vi "Average Cycle Bandwidth.vi"(10 "Decimation":u64=1, 11 "Buffer":refnum<class "Buffer.lvclass">) -> (3 "avergage cycle bandwidth":dbl format="%.0g bytes")   [LabVIEW 2017, in "DSF Core.lvlib"]
uses:
  DSF Core.lvlib
  Classes/Buffer/Buffer.lvclass
  C:/Program Files (x86)/National Instruments/LabVIEW 2017/vi.lib/NI/Memory Manager/Classes/Pointer/Pointer.lvclass
  <vilib>/NI/Memory Manager/Classes/Pointer/Pointer.lvclass/Pointer.ctl
  <vilib>/NI/Memory Manager/Classes/Pointer/Get Size.vi
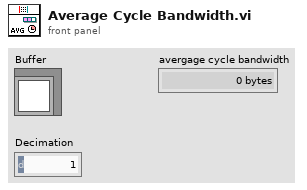
[diagram p1: front panel]
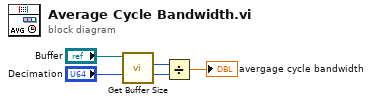
[diagram p0: block diagram]
diagram:
  n1 = call "Get Buffer Size.vi"("Buffer in"="Buffer") -> ("buffer size"=w3:u64)  [unwired: 9 in, 1 out]
  n2 = Divide(x=w3, y="Decimation") -> (x/y=→"avergage cycle bandwidth":dbl)
